vi "Convert I2C Messages & Buffer U64.vi"(8 "error in (no error)":errorcluster, 10 "STREAMING Ref":refnum<vi>, 11 "Fetched I2C Messages Ref":refnum<vi>) -> (0 "error out":errorcluster)   [LabVIEW 2025, in "I2C Bus Monitor UI.lvlib"]
uses:
  I2C Bus Monitor UI.lvlib
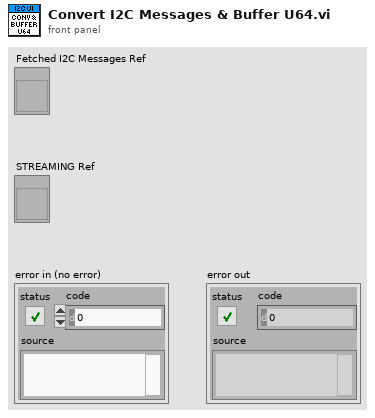
[diagram p1: front panel]
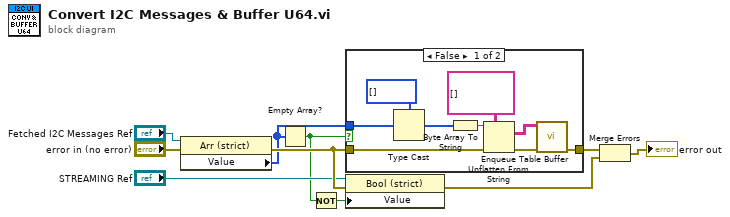
[diagram p0: block diagram]
diagram:
  n1 = property class="Arr (strict)"(reference="Fetched I2C Messages Ref", error in="error in (no error)") -> (error out=w10:errorcluster, "Value"=w7:u64[])  [unwired: 1 out]
  n2 = Empty Array?(array=w7) -> (empty?=w4:bool)
  n3 = Not(x=w4) -> (.not. x?=w3:bool)
  n4 = case shown="False" w4 {
    tunnel: w10 -> [w12 w20]
    tunnel: w7 -> [w15 _]
    tunnel: [w13 w20] -> w6
    frame False {
      n5 = Type Cast(type=u8[] [] ("unsigned byte array"), x=w15) -> (*(type *) &x=w18:u8[])
      n6 = Byte Array To String(unsigned byte array=w18) -> (string=w16:string)
      n7 = Unflatten From String(type=string[][] [] ("Fetched I2C Messages"), binary string=w16, error in (no error)=w12) -> (value=w11:string[][], error out=w14:errorcluster)  [unwired: 2 in, 1 out]
      n8 = call "Enqueue Table Buffer.vi"("error in (no error)"=w14, "Data"=w11) -> ("error out"=w13:errorcluster)  [unwired: 9 in]
    }
    frame True {
    }
  }
  n9 = property class="Bool (strict)"(reference="STREAMING Ref", error in=w10, "Value"=w3) -> (error out=w1:errorcluster)  [unwired: 1 out]
  n10 = Merge Errors(w6, w1) -> (→"error out":errorcluster)
